vi "Initialize.vi"(8 "error in (no error)":errorcluster, 9 "ID Query":bool, 10 "Reset":bool, 11 "Tektronix DMM4020 in":refnum<class "Tektronix DMM4020.lvclass">) -> (0 "error out":errorcluster, 2 "VISA resource name":refnum<visa-resource-name>, 3 "Tektronix DMM4020 out":refnum<class "Tektronix DMM4020.lvclass">)   [LabVIEW 2016, in "Generic Digital Multi Meter.lvlib" / "Tektronix DMM4020.lvlib" / "Tektronix DMM4020.lvclass"]
uses:
  Tektronix DMM4020.lvclass
  <instrlib>/Tektronix DMM4020/Tektronix DMM4020.lvlib
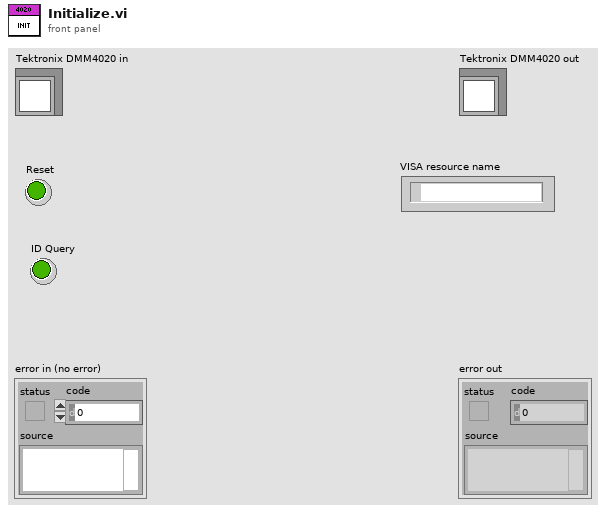
[diagram p1: front panel]
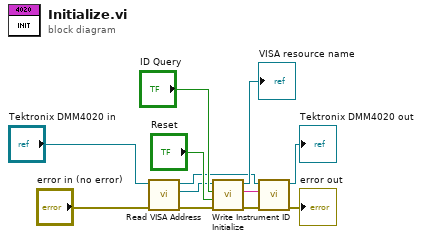
[diagram p0: block diagram]
diagram:
  n1 = call-dynamic "Read VISA Address.vi"("error in (no error)"="error in (no error)", "Generic Device in"="Tektronix DMM4020 in") -> ("error out"=w2:errorcluster, "VISA Address"=w3:refnum<visa-resource-name>, "Generic Device out"=w1:refnum<class "Tektronix DMM4020.lvclass">)  [unwired: 7 in]
  n2 = call <instrlib>:"Initialize.vi"("error in (no error)"=w2, "Reset (True)"="Reset", "ID Query (True)"="ID Query", "VISA resource name"=w3) -> ("error out"=w9:errorcluster, "ID"=w6:string, "VISA resource name out"=→"VISA resource name":refnum<visa-resource-name>)  [unwired: 5 in]
  n3 = call-dynamic "Write Instrument ID.vi"("error in (no error)"=w9, "Instrument ID"=w6, "Generic Instrument in"=w1) -> ("error out"=→"error out":errorcluster, "Generic Instrument out"=→"Tektronix DMM4020 out":refnum<class "Tektronix DMM4020.lvclass">)  [unwired: 7 in]
